vi "Dynamic Dispatch Method.vi"(8 "error in (no error)":errorcluster, 11 "class string child in":refnum<class "Child.lvclass">) -> (0 "error out":errorcluster, 2 "String":string, 3 "class string child out":refnum<class "Child.lvclass">)   [LabVIEW 2017, in "Child.lvclass"]
doc: "This is a dynamic dispatch member VI of Child .lvclass. Use this VI as a VI under test for the Dynamic Dispatch Method.lvtest test."
uses:
  Child.lvclass
  Child.lvclass/Child.ctl
panel:
  # "Overview: This is a dynamic dispatch member VI of Child.lvclass. Use this VI as a VI under test for the Dynamic Dispatch Method.lvtest test. \nRequirements: LabVIEW Full Development System, Unit Test Framework Toolkit"
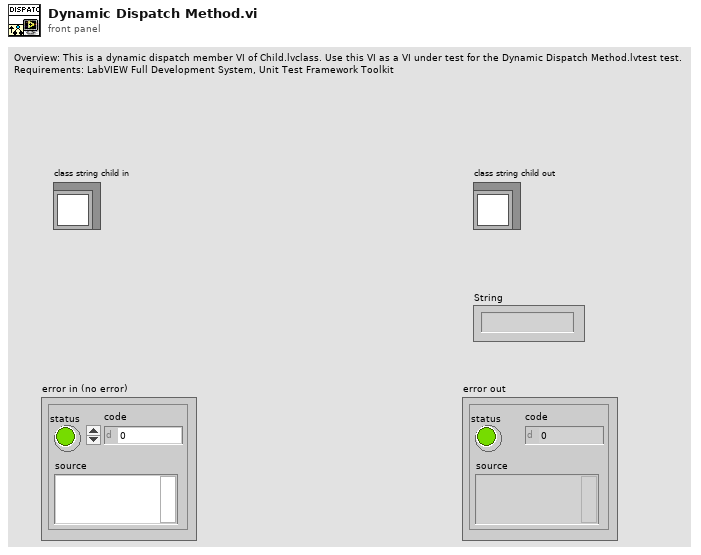
[diagram p1: front panel]
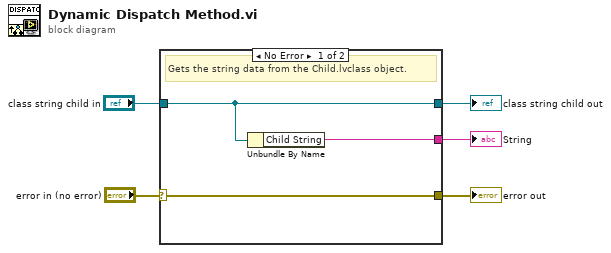
[diagram p0: block diagram]
diagram:
  n1 = case shown="No Error" "error in (no error)" {
    selector: "error in (no error)" -> [w7 w9]
    tunnel: "class string child in" -> [w6 w10]
    tunnel: [w8 _] -> w4
    tunnel: [w7 w9] -> w2
    tunnel: [w6 w10] -> w1
    frame No Error {
      # "Gets the string data from the Child.lvclass object."
      n2 = Unbundle By Name(w6) -> ("Child String"=w8:string)
    }
    frame Error {
    }
  }
  "error out" <- w2
  "class string child out" <- w1
  "String" <- w4
